vi "List Module Types.vi"() -> ()   [LabVIEW 2016]
uses:
  Module Types.ctl
panel:
  out "List of module types":string
  in  "Module type":T1
  out "Strings []":string[](array[string])
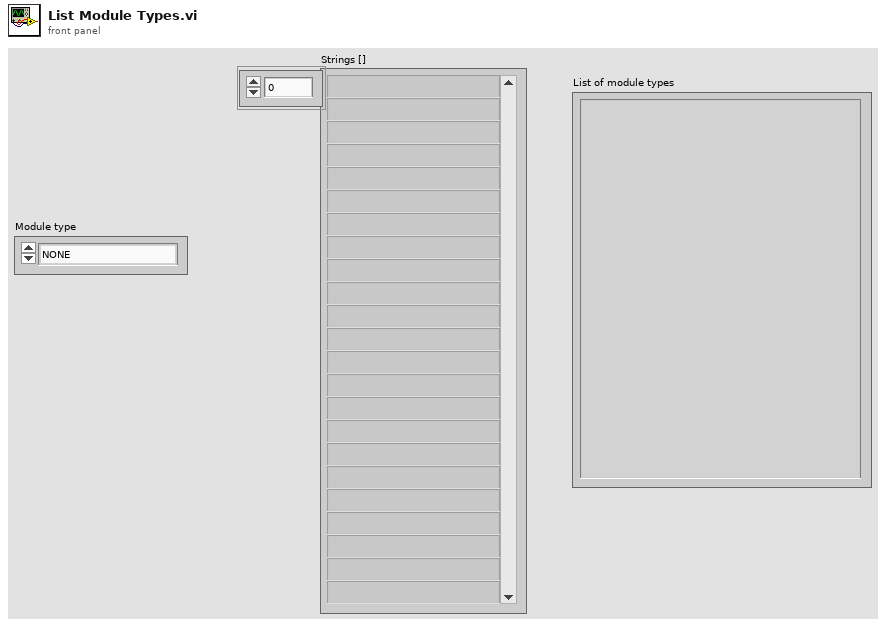
[diagram p1: front panel]
types:
  T1 = typedef "Module Types.ctl" = enum16{"NONE", "NI-DAQmx", "NI-Scope", "Red Pitaya Digitizer", "GaGe", "VISA Device", "Red Pitaya Lockin", "Monitor Controller", "Pulse Controller", "Integrate Pulse", "Lockin Processor", "File converter", "NHMFL Synthesizer", "Micron Hyperion", "Spectrum Recorder", "Resonance Detector", "TCP Communications", "Format Resonances", "Ruby Spectra", "PID Controller"}
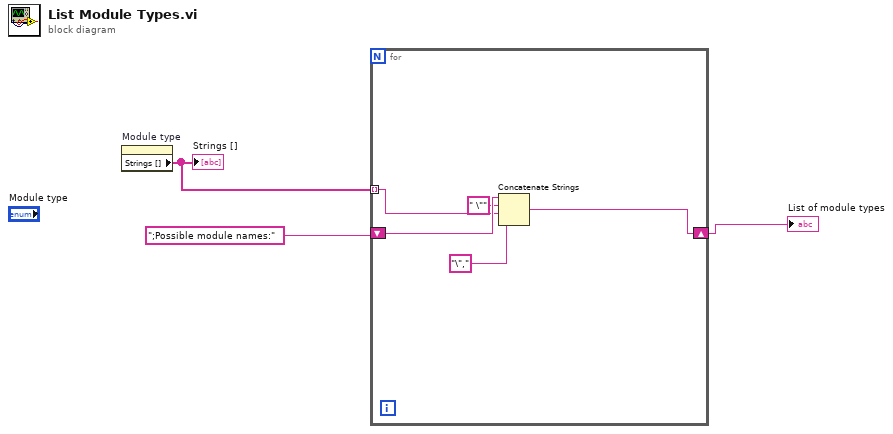
[diagram p0: block diagram]
diagram:
  n1 = property on="Module type" class="Enum (strict)"() -> ("Strings []"=w3:string[])  [unwired: 2 in, 2 out]
  "Strings []" <- w3
  n2 = for {
    tunnel: w3 -> [w7] mode=indexing
    shift-right: [w4] -> w1
    shift-left: ";Possible module names:" -> [w8]
    n3 = Concatenate Strings(w8, " \"" ("string"), w7, "\"," ("string")) -> (w4:string)
  }
  "List of module types" <- w1
